vi "HFR500 Black Box Path.vi"(2 "Channel Name String":string) -> (0 "Black Box Path":path, 1 "Black Box Folder":path)   [LabVIEW 2022 SP3]
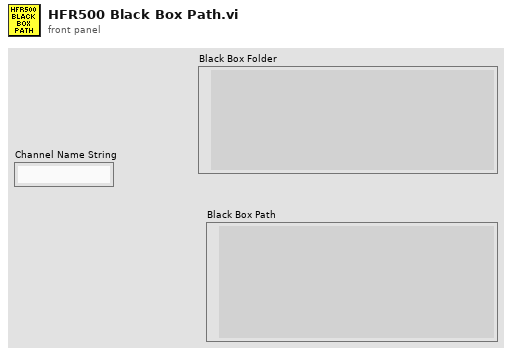
[diagram p1: front panel]
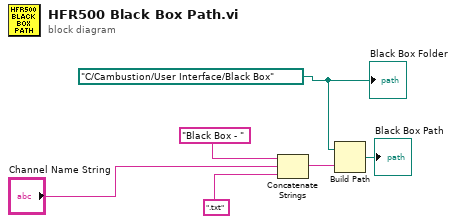
[diagram p0: block diagram]
diagram:
  w2 = path "C:/Cambustion/User Interface/Black Box" ("Path")
  n1 = Concatenate Strings("Black Box - ", "Channel Name String", ".txt" ("string")) -> (w3:string)
  n2 = Build Path(base path=w2, name or relative path=w3) -> (appended path=→"Black Box Path":path)
  "Black Box Folder" <- w2
